vi "After Launch Init.vi"(8 "error in (no error)":errorcluster, 11 "HIJ Vision Camera App In":refnum<class "HIJ Vision Camera App.lvclass">) -> (0 "error out":errorcluster, 3 "HIJ Vision Camera App Out":refnum<class "HIJ Vision Camera App.lvclass">)   [LabVIEW 2020, in "HIJ Vision Camera App.lvlib" / "HIJ Vision Camera App.lvclass"]
uses:
  HIJ Vision Camera App.lvclass
  C:/Program Files (x86)/National Instruments/LabVIEW 2020/vi.lib/ActorFramework/Actor/Actor.lvclass
  C:/POLARIS Programme/POLARIS-AS-3-Cams/Submodules/HIJ Vision/Application Base Actors/HIJ Vision Application/HIJ Vision Application/HIJ Vision Application.lvclass
  HIJ Vision Camera App Messages/New Image Msg/New Image Msg.lvclass
  C:/POLARIS Programme/POLARIS-AS-3-Cams/Submodules/HIJ Vision/Camera Actors/Camera Actor/Camera Actor Messages/New Image Msg/New Image Msg.lvclass
  HIJ Vision Camera App.lvclass/HIJ Vision Camera App.ctl
  <vilib>/ActorFramework/Actor/Actor.lvclass/Actor.ctl
  <vilib>/ActorFramework/Message Enqueuer/Message Enqueuer.lvclass/Message Enqueuer.ctl
  Camera Actors/Camera Actor/Camera Actor Messages/Write Receiver Params Msg/Write Receiver Params Msg.lvclass/Write Receiver Params Msg.ctl
  HIJ Vision Application/HIJ Vision Application/Read Display Enq.vi
  <vilib>/ActorFramework/Message Enqueuer/Init from Existing Queue.vi
  <vilib>/ActorFramework/Message Enqueuer/Enqueue.vi
  Camera Actors/Camera Actor/Camera Actor Messages/Write Receiver Params Msg/Write Receiver Params Msg.lvclass
  C:/Program Files (x86)/National Instruments/LabVIEW 2020/vi.lib/ActorFramework/Message/Message.lvclass
  <vilib>/ActorFramework/Message Priority Queue/Priority Enqueue.vi
  HIJ Vision Application/HIJ Vision Application/HIJ Vision Application.lvclass
  <vilib>/ActorFramework/Message Enqueuer/Message Enqueuer.lvclass
  <vilib>/ActorFramework/Actor/Actor.lvclass
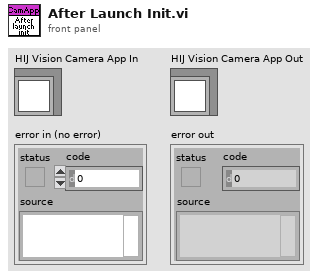
[diagram p1: front panel]
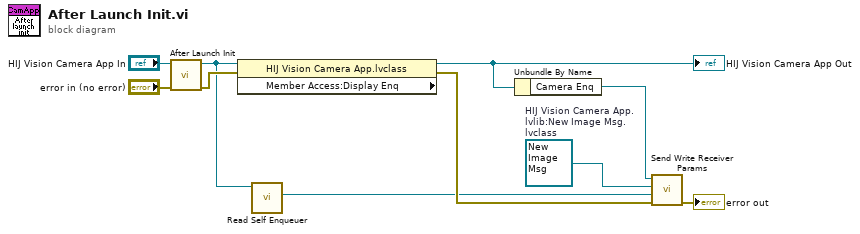
[diagram p0: block diagram]
diagram:
  w1 = refnum<class "New Image Msg.lvclass"> refnum  # HIJ Vision Camera App.lvlib:New Image Msg.lvclass
  n1 = call-parent "After Launch Init.vi"("error in (no error)"="error in (no error)", "HIJ Vision Application in"="HIJ Vision Camera App In") -> ("error out"=w6:errorcluster, "HIJ Vision Application out"=w3:refnum<class "HIJ Vision Camera App.lvclass">)  [unwired: 8 in]
  n2 = property class="HIJ Vision Camera App.lvclass" props=["Member Access:Display Enq"](reference=w3, error in=w6) -> (reference out=w8:refnum<class "HIJ Vision Camera App.lvclass">, error out=w5:errorcluster)  [unwired: 1 out]
  "HIJ Vision Camera App Out" <- w8
  n3 = call <vilib>:"Read Self Enqueuer.vi"("Actor"=w3) -> ("Self Enqueuer"=w2:refnum<class "Message Enqueuer.lvclass">)  [unwired: 10 in]
  n4 = Unbundle By Name(w8) -> ("Camera Enq"=w7:refnum<class "Message Enqueuer.lvclass">)
  n5 = call "Send Write Receiver Params.vi"("error in (no error)"=w5, "Image Receiver"=w2, "New Image Msg"=w1, "Message Enqueuer"=w7) -> ("error out"=→"error out":errorcluster)  [unwired: 6 in, 1 out]
